vi "输入数据解析.vi"(0 "单个参数补充":dbl, 1 "从板号":dbl=1.0, 2 "主板二维码":string="BNET01", 3 "从板二维码":string="BNET01", 5 "主板引用":refnum<vi>, 7 "从板引用":refnum<vi>, 9 "主板选项":string="三级故障阀值", 11 "枚举":enum16{"主板", "从板"}(ring), 12 "快换":bool caption="快换写入") -> (4 "输出数组":dbl[][](array[numeric]), 6 "数组长度":dbl[](array[numeric]), 8 "循环次数":i32, 10 "命令":u32, 14 "名称":string[](array[string]), 15 "命令序号":u32[](array[numeric]))   [LabVIEW 2013] (continued)
                n3199 = Build Array(w8273, w8271) -> (w8272:dbl[])
              }
              frame 11 {
                # "单组温度不均衡"
                n3200 = disable-structure shown="启用" {
                  disable-tunnel: [w8288 255 ("高字节1")] -> w8284
                  disable-tunnel: w8282 -> [w8286 _]
                  frame Disabled {
                    n3201 = Unbundle By Name(w8286) -> ("单组温度不均衡"=w8285:dbl)
                    n3202 = call "输入分辨率计算-EV05.vi"("1字节?"=TRUE, "数值"=w8285, "偏移量"=0.0, "分辨率"=1.0) -> ("高字节1"=w8288:dbl)  [unwired: 1 in, 6 out]
                  }
                  frame Enabled {
                  }
                }
                n3203 = Build Array(w8284) -> (w8283:i32[])
              }
              frame 12 {
                n3204 = Unbundle By Name(w8296) -> ("SOC过高"=w8295:dbl)
                n3205 = call "输入分辨率计算-EV05.vi"("1字节?"=FALSE, "数值"=w8295, "偏移量"=0.0, "分辨率"=0.1) -> ("低字节"=w8297:dbl, "高字节1"=w8298:dbl)  [unwired: 1 in, 5 out]
                n3206 = call "二进制解析-8.6.vi"("索引"=4, "数值"=w8298) -> ("低位子数组"=w8301:i32[])  [unwired: 3 out]
                n3207 = call "二进制解析-8.6.vi"("索引"=4, "数值"=w8297) -> ("低位子数组"=w8293:i32[], "高位子数组"=w8300:i32[])  [unwired: 2 out]
                n3208 = Insert Into Array(array=w8301, new element=w8300) -> (w8299:i32[])  [unwired: 1 in]
                n3209 = call "数值二进制转十进制-8.6.vi"("子数组"=w8299) -> ("十进制数值"=w8294:i32)  [unwired: 4 out]
                n3210 = disable-structure shown="启用" {
                  disable-tunnel: w8294 -> [w8309 _]
                  disable-tunnel: [w8309 255 ("高字节1")] -> w8292
                  disable-tunnel: [w8308 i32[] [] ("低位子数组 28")] -> _
                  disable-tunnel: w8293 -> [w8308 _]
                  frame Disabled {
                  }
                  frame Enabled {
                  }
                }
                n3211 = Build Array(w8292, w8292) -> (w8305:i32[])
              }
              frame 13 {
                # "SOC过低"
                n3212 = Unbundle By Name(w8317) -> ("SOC过低"=w8316:dbl)
                n3213 = call "输入分辨率计算-EV05.vi"("1字节?"=FALSE, "数值"=w8316, "偏移量"=0.0, "分辨率"=0.1) -> ("低字节"=w8314:dbl, "高字节1"=w8315:dbl)  [unwired: 1 in, 5 out]
                n3214 = call "二进制解析-8.6.vi"("索引"=4, "数值"=w8315) -> ("低位子数组"=w8313:i32[])  [unwired: 3 out]
                n3215 = disable-structure shown="启用" {
                  disable-tunnel: w8314 -> [w8324 _]
                  disable-tunnel: [w8324 255 ("高字节1")] -> w8312
                  disable-tunnel: w8313 -> [w8323 _]
                  disable-tunnel: [w8323 i32[] [] ("低位子数组")] -> _
                  frame Disabled {
                    (unwired) i32[] [] ("低位子数组 4")
                  }
                  frame Enabled {
                  }
                }
                n3216 = Build Array(w8312, w8312) -> (w8320:i32[])
              }
              frame 14 {
                # "内阻过大"
                n3217 = disable-structure shown="启用" {
                  disable-tunnel: w8329 -> [w8334 _]
                  disable-tunnel: [w8330 255 ("高字节1")] -> w8327
                  frame Disabled {
                    n3218 = Unbundle By Name(w8334) -> ("内阻过大"=w8333:dbl)
                    n3219 = call "输入分辨率计算-EV05.vi"("1字节?"=TRUE, "数值"=w8333, "分辨率"=0.1) -> ("高字节1"=w8330:dbl)  [unwired: 2 in, 6 out]
                  }
                  frame Enabled {
                  }
                }
                n3220 = Build Array(w8327) -> (w8328:i32[])
              }
              frame 15 {
                # "极柱温度过高"
                n3221 = disable-structure shown="启用" {
                  disable-tunnel: w8338 -> [w8344 _]
                  disable-tunnel: [w8340 255 ("高字节1")] -> w8336
                  frame Disabled {
                    n3222 = Unbundle By Name(w8344) -> ("极柱温度过高"=w8343:dbl)
                    n3223 = call "输入分辨率计算-EV05.vi"("1字节?"=TRUE, "数值"=w8343, "偏移量"=-40.0, "分辨率"=1.0) -> ("高字节1"=w8340:dbl)  [unwired: 1 in, 6 out]
                  }
                  frame Enabled {
                  }
                }
                n3224 = Build Array(w8336) -> (w8337:i32[])
              }
              frame 16 {
                # "SOH过低"
                n3225 = disable-structure shown="启用" {
                  disable-tunnel: [w8361 w8369] -> w8348
                  disable-tunnel: w8347 -> [w8358 _]
                  disable-tunnel: [w8350 w8369] -> w8346
                  frame Disabled {
                    n3226 = Unbundle By Name(w8358) -> ("SOH过低"=w8357:dbl)
                    n3227 = call "输入分辨率计算-EV05.vi"("1字节?"=FALSE, "数值"=w8357, "偏移量"=0.0, "分辨率"=0.1) -> ("低字节"=w8359:dbl, "高字节1"=w8360:dbl)  [unwired: 1 in, 5 out]
                    n3228 = call "二进制解析-8.6.vi"("索引"=4, "数值"=w8360) -> ("低位子数组"=w8363:i32[])  [unwired: 3 out]
                    n3229 = call "二进制解析-8.6.vi"("索引"=4, "数值"=w8359) -> ("低位子数组"=w8352:i32[], "高位子数组"=w8362:i32[])  [unwired: 2 out]
                    n3230 = call "二进制解析-8.6.vi"("索引"=4, "数值"=0) -> ("低位子数组"=w8353:i32[])  [unwired: 3 out]
                    n3231 = Insert Into Array(array=w8363, new element=w8362) -> (w8356:i32[])  [unwired: 1 in]
                    n3232 = Insert Into Array(array=w8352, new element=w8353) -> (w8351:i32[])  [unwired: 1 in]
                    n3233 = call "数值二进制转十进制-8.6.vi"("子数组"=w8356) -> ("十进制数值"=w8361:i32)  [unwired: 4 out]
                    n3234 = call "数值二进制转十进制-8.6.vi"("子数组"=w8351) -> ("十进制数值"=w8350:i32)  [unwired: 4 out]
                  }
                  frame Enabled {
                    w8369 = 255 ("高字节1")
                  }
                }
                n3235 = Build Array(w8348, w8346) -> (w8349:i32[])
              }
            }
            n3236 = Insert Into Array(array=w8154, new element=w8155) -> (w8153:dbl[])  [unwired: 1 in]
          }
          n3237 = Build Array(w8150) -> (w8149:dbl[][])
          n3238 = Build Array("二级故障阀值") -> (w8140:string[])
        }
        frame "放电电流过高(3)" {
          n3239 = Unbundle By Name(w8375) -> ("一级故障 3"=w8376:refnum<vi>)
          n3240 = property class="Clust (严格)"(reference=w8376) -> ("Value"=w8374:T4)  [unwired: 1 in, 2 out]
          n3241 = for {
            N: 17 -> [_]
            tunnel: w8374 -> [w8386]
            shift-right: [w8383] -> w8380
            shift-left: dbl[] [] -> [w8384]
            i -> [w8387]
            n3242 = case shown="14" w8387 {
              tunnel: w8386 -> [w8388 w8399 w8410 w8420 w8430 w8440 w8452 w8464 w8476 w8488 w8500 w8512 w8526 w8547 w8559 w8568 w8577]
              tunnel: [w8389 w8400 w8411 w8421 w8431 w8442 w8454 w8466 w8478 w8490 w8502 w8513 w8535 w8550 w8558 w8567 w8579] -> w8385
              frame 0, Default {
                # "总电压过高"
                n3243 = disable-structure shown="启用" {
                  disable-tunnel: [w8395 w8398] -> w8391
                  disable-tunnel: [w8394 w8398] -> w8390
                  disable-tunnel: w8388 -> [w8393 _]
                  frame Disabled {
                    n3244 = Unbundle By Name(w8393) -> ("总电压过高"=w8392:dbl)
                    n3245 = call "输入分辨率计算-EV05.vi"("1字节?"=FALSE, "数值"=w8392, "分辨率"=0.1) -> ("低字节"=w8395:dbl, "高字节1"=w8394:dbl)  [unwired: 2 in, 5 out]
                  }
                  frame Enabled {
                    w8398 = 255 ("高字节1")
                  }
                }
                n3246 = Build Array(w8390, w8391) -> (w8389:i32[])
              }
              frame 1 {
                # "总电压过低"
                n3247 = disable-structure shown="启用" {
                  disable-tunnel: [w8406 w8409] -> w8402
                  disable-tunnel: [w8405 w8409] -> w8401
                  disable-tunnel: w8399 -> [w8404 _]
                  frame Disabled {
                    n3248 = Unbundle By Name(w8404) -> ("总电压过低"=w8403:dbl)
                    n3249 = call "输入分辨率计算-EV05.vi"("1字节?"=FALSE, "数值"=w8403, "分辨率"=0.1) -> ("低字节"=w8406:dbl, "高字节1"=w8405:dbl)  [unwired: 2 in, 5 out]
                  }
                  frame Enabled {
                    w8409 = 255 ("高字节1")
                  }
                }
                n3250 = Build Array(w8401, w8402) -> (w8400:i32[])
              }
              frame 2 {
                # "温度过高"
                n3251 = disable-structure shown="启用" {
                  disable-tunnel: [w8416 255 ("高字节1")] -> w8412
                  disable-tunnel: w8410 -> [w8414 _]
                  frame Disabled {
                    n3252 = Unbundle By Name(w8414) -> ("温度过高"=w8413:dbl)
                    n3253 = call "输入分辨率计算-EV05.vi"("1字节?"=TRUE, "数值"=w8413, "偏移量"=-40.0, "分辨率"=1.0) -> ("高字节1"=w8416:dbl)  [unwired: 1 in, 6 out]
                  }
                  frame Enabled {
                  }
                }
                n3254 = Build Array(w8412) -> (w8411:i32[])
              }
              frame 3 {
                # "温度过低"
                n3255 = disable-structure shown="启用" {
                  disable-tunnel: [w8426 255 ("高字节1")] -> w8422
                  disable-tunnel: w8420 -> [w8424 _]
                  frame Disabled {
                    n3256 = Unbundle By Name(w8424) -> ("温度过低"=w8423:dbl)
                    n3257 = call "输入分辨率计算-EV05.vi"("1字节?"=TRUE, "数值"=w8423, "偏移量"=-40.0, "分辨率"=1.0) -> ("高字节1"=w8426:dbl)  [unwired: 1 in, 6 out]
                  }
                  frame Enabled {
                  }
                }
                n3258 = Build Array(w8422) -> (w8421:i32[])
              }
              frame 4 {
                # "整组温度不均衡"
                n3259 = disable-structure shown="启用" {
                  disable-tunnel: [w8436 255 ("高字节1")] -> w8432
                  disable-tunnel: w8430 -> [w8434 _]
                  frame Disabled {
                    n3260 = Unbundle By Name(w8434) -> ("整组温度不均衡"=w8433:dbl)
                    n3261 = call "输入分辨率计算-EV05.vi"("1字节?"=TRUE, "数值"=w8433, "偏移量"=0.0, "分辨率"=1.0) -> ("高字节1"=w8436:dbl)  [unwired: 1 in, 6 out]
                  }
                  frame Enabled {
                  }
                }
                n3262 = Build Array(w8432) -> (w8431:i32[])
              }
              frame 5 {
                # "单组电压不均衡"
                n3263 = disable-structure shown="启用" {
                  disable-tunnel: [w8448 w8451] -> w8443
                  disable-tunnel: [w8446 w8451] -> w8441
                  disable-tunnel: w8440 -> [w8445 _]
                  frame Disabled {
                    n3264 = Unbundle By Name(w8445) -> ("单组电压不均衡"=w8444:dbl)
                    n3265 = call "输入分辨率计算-EV05.vi"("1字节?"=FALSE, "数值"=w8444, "偏移量"=0.0, "分辨率"=0.001) -> ("低字节"=w8446:dbl, "高字节1"=w8448:dbl)  [unwired: 1 in, 5 out]
                  }
                  frame Enabled {
                    w8451 = 255 ("高字节1")
                  }
                }
                n3266 = Build Array(w8443, w8441) -> (w8442:i32[])
              }
              frame 6 {
                # "整组电压不均衡"
                n3267 = disable-structure shown="启用" {
                  disable-tunnel: [w8460 w8463] -> w8455
                  disable-tunnel: [w8458 w8463] -> w8453
                  disable-tunnel: w8452 -> [w8457 _]
                  frame Disabled {
                    n3268 = Unbundle By Name(w8457) -> ("整组电压不均衡"=w8456:dbl)
                    n3269 = call "输入分辨率计算-EV05.vi"("1字节?"=FALSE, "数值"=w8456, "偏移量"=0.0, "分辨率"=0.001) -> ("低字节"=w8458:dbl, "高字节1"=w8460:dbl)  [unwired: 1 in, 5 out]
                  }
                  frame Enabled {
                    w8463 = 255 ("高字节1")
                  }
                }
                n3270 = Build Array(w8455, w8453) -> (w8454:i32[])
              }
              frame 7 {
                # "单体电压过高"
                n3271 = disable-structure shown="启用" {
                  disable-tunnel: [w8472 w8475] -> w8467
                  disable-tunnel: [w8470 w8475] -> w8465
                  disable-tunnel: w8464 -> [w8469 _]
                  frame Disabled {
                    n3272 = Unbundle By Name(w8469) -> ("单体电压过高"=w8468:dbl)
                    n3273 = call "输入分辨率计算-EV05.vi"("1字节?"=FALSE, "数值"=w8468, "偏移量"=0.0, "分辨率"=0.001) -> ("低字节"=w8470:dbl, "高字节1"=w8472:dbl)  [unwired: 1 in, 5 out]
                  }
                  frame Enabled {
                    w8475 = 255 ("高字节1")
                  }
                }
                n3274 = Build Array(w8467, w8465) -> (w8466:i32[])
              }
              frame 8 {
                # "单体电压过低"
                n3275 = disable-structure shown="启用" {
                  disable-tunnel: [w8484 w8487] -> w8479
                  disable-tunnel: [w8482 w8487] -> w8477
                  disable-tunnel: w8476 -> [w8481 _]
                  frame Disabled {
                    n3276 = Unbundle By Name(w8481) -> ("单体电压过低"=w8480:dbl)
                    n3277 = call "输入分辨率计算-EV05.vi"("1字节?"=FALSE, "数值"=w8480, "偏移量"=0.0, "分辨率"=0.001) -> ("低字节"=w8482:dbl, "高字节1"=w8484:dbl)  [unwired: 1 in, 5 out]
                  }
                  frame Enabled {
                    w8487 = 255 ("高字节1")
                  }
                }
                n3278 = Build Array(w8479, w8477) -> (w8478:i32[])
              }
              frame 9 {
                # "充电电流过高"
                n3279 = disable-structure shown="启用" {
                  disable-tunnel: [w8496 w8499] -> w8491
                  disable-tunnel: [w8494 w8499] -> w8489
                  disable-tunnel: w8488 -> [w8493 _]
                  frame Disabled {
                    n3280 = Unbundle By Name(w8493) -> ("充电电流过高"=w8492:dbl)
                    n3281 = call "输入分辨率计算-EV05.vi"("1字节?"=FALSE, "数值"=w8492, "偏移量"=-3000.0, "分辨率"=0.1) -> ("低字节"=w8494:dbl, "高字节1"=w8496:dbl)  [unwired: 1 in, 5 out]
                  }
                  frame Enabled {
                    w8499 = 255 ("高字节1")
                  }
                }
                n3282 = Build Array(w8491, w8489) -> (w8490:i32[])
              }
              frame 10 {
                # "放电电流过高"
                n3283 = disable-structure shown="启用" {
                  disable-tunnel: [w8508 w8511] -> w8503
                  disable-tunnel: [w8506 w8511] -> w8501
                  disable-tunnel: w8500 -> [w8505 _]
                  frame Enabled {
                    n3284 = Unbundle By Name(w8505) -> ("放电电流过高"=w8504:dbl)
                    n3285 = call "输入分辨率计算-EV05.vi"("1字节?"=FALSE, "数值"=w8504, "偏移量"=0.0, "分辨率"=0.1) -> ("低字节"=w8506:dbl, "高字节1"=w8508:dbl)  [unwired: 1 in, 5 out]
                  }
                  frame Disabled {
                    w8511 = 255 ("高字节1")
                  }
                }
                n3286 = Build Array(w8503, w8501) -> (w8502:dbl[])
              }
              frame 11 {
                # "单组温度不均衡"
                n3287 = disable-structure shown="启用" {
                  disable-tunnel: [w8518 255 ("高字节1")] -> w8514
                  disable-tunnel: w8512 -> [w8516 _]
                  frame Disabled {
                    n3288 = Unbundle By Name(w8516) -> ("单组温度不均衡"=w8515:dbl)
                    n3289 = call "输入分辨率计算-EV05.vi"("1字节?"=TRUE, "数值"=w8515, "偏移量"=0.0, "分辨率"=1.0) -> ("高字节1"=w8518:dbl)  [unwired: 1 in, 6 out]
                  }
                  frame Enabled {
                  }
                }
                n3290 = Build Array(w8514) -> (w8513:i32[])
              }
              frame 12 {
                # "SOC过高"
                n3291 = Unbundle By Name(w8526) -> ("SOC过高"=w8525:dbl)
                n3292 = call "输入分辨率计算-EV05.vi"("1字节?"=FALSE, "数值"=w8525, "偏移量"=0.0, "分辨率"=0.1) -> ("低字节"=w8527:dbl, "高字节1"=w8528:dbl)  [unwired: 1 in, 5 out]
                n3293 = call "二进制解析-8.6.vi"("索引"=4, "数值"=w8528) -> ("低位子数组"=w8531:i32[])  [unwired: 3 out]
                n3294 = call "二进制解析-8.6.vi"("索引"=4, "数值"=w8527) -> ("低位子数组"=w8523:i32[], "高位子数组"=w8530:i32[])  [unwired: 2 out]
                n3295 = Insert Into Array(array=w8531, new element=w8530) -> (w8529:i32[])  [unwired: 1 in]
                n3296 = call "数值二进制转十进制-8.6.vi"("子数组"=w8529) -> ("十进制数值"=w8524:i32)  [unwired: 4 out]
                n3297 = disable-structure shown="启用" {
                  disable-tunnel: w8524 -> [w8539 _]
                  disable-tunnel: [w8539 255 ("高字节1")] -> w8522
                  disable-tunnel: [w8538 i32[] [] ("低位子数组 28")] -> _
                  disable-tunnel: w8523 -> [w8538 _]
                  frame Disabled {
                  }
                  frame Enabled {
                  }
                }
                n3298 = Build Array(w8522, w8522) -> (w8535:i32[])
              }
              frame 13 {
                # "SOC过低"
                n3299 = Unbundle By Name(w8547) -> ("SOC过低"=w8546:dbl)
                n3300 = call "输入分辨率计算-EV05.vi"("1字节?"=FALSE, "数值"=w8546, "偏移量"=0.0, "分辨率"=0.1) -> ("低字节"=w8544:dbl, "高字节1"=w8545:dbl)  [unwired: 1 in, 5 out]
                n3301 = call "二进制解析-8.6.vi"("索引"=4, "数值"=w8545) -> ("低位子数组"=w8543:i32[])  [unwired: 3 out]
                n3302 = disable-structure shown="启用" {
                  disable-tunnel: w8544 -> [w8554 _]
                  disable-tunnel: [w8554 255 ("高字节1")] -> w8542
                  disable-tunnel: w8543 -> [w8553 _]
                  disable-tunnel: [w8553 i32[] [] ("低位子数组")] -> _
                  frame Disabled {
                    (unwired) i32[] [] ("低位子数组 4")
                  }
                  frame Enabled {
                  }
                }
                n3303 = Build Array(w8542, w8542) -> (w8550:i32[])
              }
              frame 14 {
                # "内阻过大"
                n3304 = disable-structure shown="启用" {
                  disable-tunnel: w8559 -> [w8564 _]
                  disable-tunnel: [w8560 255 ("高字节1")] -> w8557
                  frame Disabled {
                    n3305 = Unbundle By Name(w8564) -> ("内阻过大"=w8563:dbl)
                    n3306 = call "输入分辨率计算-EV05.vi"("1字节?"=TRUE, "数值"=w8563, "分辨率"=0.1) -> ("高字节1"=w8560:dbl)  [unwired: 2 in, 6 out]
                  }
                  frame Enabled {
                  }
                }
                n3307 = Build Array(w8557) -> (w8558:i32[])
              }
              frame 15 {
                # "极柱温度过高"
                n3308 = disable-structure shown="启用" {
                  disable-tunnel: w8568 -> [w8574 _]
                  disable-tunnel: [w8570 255 ("高字节1")] -> w8566
                  frame Disabled {
                    n3309 = Unbundle By Name(w8574) -> ("极柱温度过高"=w8573:dbl)
                    n3310 = call "输入分辨率计算-EV05.vi"("1字节?"=TRUE, "数值"=w8573, "偏移量"=-40.0, "分辨率"=1.0) -> ("高字节1"=w8570:dbl)  [unwired: 1 in, 6 out]
                  }
                  frame Enabled {
                  }
                }
                n3311 = Build Array(w8566) -> (w8567:i32[])
              }
              frame 16 {
                # "SOH过低"
                n3312 = disable-structure shown="启用" {
                  disable-tunnel: [w8591 w8599] -> w8578
                  disable-tunnel: w8577 -> [w8588 _]
                  disable-tunnel: [w8580 w8599] -> w8576
                  frame Disabled {
                    n3313 = Unbundle By Name(w8588) -> ("SOH过低"=w8587:dbl)
                    n3314 = call "输入分辨率计算-EV05.vi"("1字节?"=FALSE, "数值"=w8587, "偏移量"=0.0, "分辨率"=0.1) -> ("低字节"=w8589:dbl, "高字节1"=w8590:dbl)  [unwired: 1 in, 5 out]
                    n3315 = call "二进制解析-8.6.vi"("索引"=4, "数值"=w8590) -> ("低位子数组"=w8593:i32[])  [unwired: 3 out]
                    n3316 = call "二进制解析-8.6.vi"("索引"=4, "数值"=w8589) -> ("低位子数组"=w8582:i32[], "高位子数组"=w8592:i32[])  [unwired: 2 out]
                    n3317 = call "二进制解析-8.6.vi"("索引"=4, "数值"=0) -> ("低位子数组"=w8583:i32[])  [unwired: 3 out]
                    n3318 = Insert Into Array(array=w8593, new element=w8592) -> (w8586:i32[])  [unwired: 1 in]
                    n3319 = Insert Into Array(array=w8582, new element=w8583) -> (w8581:i32[])  [unwired: 1 in]
                    n3320 = call "数值二进制转十进制-8.6.vi"("子数组"=w8586) -> ("十进制数值"=w8591:i32)  [unwired: 4 out]
                    n3321 = call "数值二进制转十进制-8.6.vi"("子数组"=w8581) -> ("十进制数值"=w8580:i32)  [unwired: 4 out]
                  }
                  frame Enabled {
                    w8599 = 255 ("高字节1")
                  }
                }
                n3322 = Build Array(w8578, w8576) -> (w8579:i32[])
              }
            }
            n3323 = Insert Into Array(array=w8384, new element=w8385) -> (w8383:dbl[])  [unwired: 1 in]
          }
          n3324 = Build Array(w8380) -> (w8379:dbl[][])
          n3325 = Build Array("三级故障阀值") -> (w8370:string[])
        }
        frame "单组温度不均衡" {
          n3326 = Unbundle By Name(w8605) -> ("一级故障"=w8606:refnum<vi>)
          n3327 = property class="Clust (严格)"(reference=w8606) -> ("Value"=w8604:T4)  [unwired: 1 in, 2 out]
          n3328 = for {
            N: 17 -> [_]
            tunnel: w8604 -> [w8616]
            shift-right: [w8613] -> w8610
            shift-left: dbl[] [] -> [w8614]
            i -> [w8617]
            n3329 = case shown="11" w8617 {
              tunnel: w8616 -> [w8618 w8629 w8640 w8650 w8660 w8670 w8682 w8694 w8706 w8718 w8730 w8742 w8755 w8776 w8788 w8797 w8806]
              tunnel: [w8619 w8630 w8641 w8651 w8661 w8672 w8684 w8696 w8708 w8720 w8732 w8743 w8764 w8779 w8787 w8796 w8808] -> w8615
              frame 0, Default {
                # "总电压过高"
                n3330 = disable-structure shown="启用" {
                  disable-tunnel: [w8625 w8628] -> w8621
                  disable-tunnel: [w8624 w8628] -> w8620
                  disable-tunnel: w8618 -> [w8623 _]
                  frame Disabled {
                    n3331 = Unbundle By Name(w8623) -> ("总电压过高"=w8622:dbl)
                    n3332 = call "输入分辨率计算-EV05.vi"("1字节?"=FALSE, "数值"=w8622, "分辨率"=0.1) -> ("低字节"=w8625:dbl, "高字节1"=w8624:dbl)  [unwired: 2 in, 5 out]
                  }
                  frame Enabled {
                    w8628 = 255 ("高字节1")
                  }
                }
                n3333 = Build Array(w8620, w8621) -> (w8619:i32[])
              }
              frame 1 {
                # "总电压过低"
                n3334 = disable-structure shown="启用" {
                  disable-tunnel: [w8636 w8639] -> w8632
                  disable-tunnel: [w8635 w8639] -> w8631
                  disable-tunnel: w8629 -> [w8634 _]
                  frame Disabled {
                    n3335 = Unbundle By Name(w8634) -> ("总电压过低"=w8633:dbl)
                    n3336 = call "输入分辨率计算-EV05.vi"("1字节?"=FALSE, "数值"=w8633, "分辨率"=0.1) -> ("低字节"=w8636:dbl, "高字节1"=w8635:dbl)  [unwired: 2 in, 5 out]
                  }
                  frame Enabled {
                    w8639 = 255 ("高字节1")
                  }
                }
                n3337 = Build Array(w8631, w8632) -> (w8630:i32[])
              }
              frame 2 {
                # "温度过高"
                n3338 = disable-structure shown="启用" {
                  disable-tunnel: [w8646 255 ("高字节1")] -> w8642
                  disable-tunnel: w8640 -> [w8644 _]
                  frame Disabled {
                    n3339 = Unbundle By Name(w8644) -> ("温度过高"=w8643:dbl)
                    n3340 = call "输入分辨率计算-EV05.vi"("1字节?"=TRUE, "数值"=w8643, "偏移量"=-40.0, "分辨率"=1.0) -> ("高字节1"=w8646:dbl)  [unwired: 1 in, 6 out]
                  }
                  frame Enabled {
                  }
                }
                n3341 = Build Array(w8642) -> (w8641:i32[])
              }
              frame 3 {
                # "温度过低"
                n3342 = disable-structure shown="启用" {
                  disable-tunnel: [w8656 255 ("高字节1")] -> w8652
                  disable-tunnel: w8650 -> [w8654 _]
                  frame Disabled {
                    n3343 = Unbundle By Name(w8654) -> ("温度过低"=w8653:dbl)
                    n3344 = call "输入分辨率计算-EV05.vi"("1字节?"=TRUE, "数值"=w8653, "偏移量"=-40.0, "分辨率"=1.0) -> ("高字节1"=w8656:dbl)  [unwired: 1 in, 6 out]
                  }
                  frame Enabled {
                  }
                }
                n3345 = Build Array(w8652) -> (w8651:i32[])
              }
              frame 4 {
                # "整组温度不均衡"
                n3346 = disable-structure shown="启用" {
                  disable-tunnel: [w8666 255 ("高字节1")] -> w8662
                  disable-tunnel: w8660 -> [w8664 _]
                  frame Disabled {
                    n3347 = Unbundle By Name(w8664) -> ("整组温度不均衡"=w8663:dbl)
                    n3348 = call "输入分辨率计算-EV05.vi"("1字节?"=TRUE, "数值"=w8663, "偏移量"=0.0, "分辨率"=1.0) -> ("高字节1"=w8666:dbl)  [unwired: 1 in, 6 out]
                  }
                  frame Enabled {
                  }
                }
                n3349 = Build Array(w8662) -> (w8661:i32[])
              }
              frame 5 {
                # "单组电压不均衡"
                n3350 = disable-structure shown="启用" {
                  disable-tunnel: [w8678 w8681] -> w8673
                  disable-tunnel: [w8676 w8681] -> w8671
                  disable-tunnel: w8670 -> [w8675 _]
                  frame Disabled {
                    n3351 = Unbundle By Name(w8675) -> ("单组电压不均衡"=w8674:dbl)
                    n3352 = call "输入分辨率计算-EV05.vi"("1字节?"=FALSE, "数值"=w8674, "偏移量"=0.0, "分辨率"=0.001) -> ("低字节"=w8676:dbl, "高字节1"=w8678:dbl)  [unwired: 1 in, 5 out]
                  }
                  frame Enabled {
                    w8681 = 255 ("高字节1")
                  }
                }
                n3353 = Build Array(w8673, w8671) -> (w8672:i32[])
              }
              frame 6 {
                # "整组电压不均衡"
                n3354 = disable-structure shown="启用" {
                  disable-tunnel: [w8690 w8693] -> w8685
                  disable-tunnel: [w8688 w8693] -> w8683
                  disable-tunnel: w8682 -> [w8687 _]
                  frame Disabled {
                    n3355 = Unbundle By Name(w8687) -> ("整组电压不均衡"=w8686:dbl)
                    n3356 = call "输入分辨率计算-EV05.vi"("1字节?"=FALSE, "数值"=w8686, "偏移量"=0.0, "分辨率"=0.001) -> ("低字节"=w8688:dbl, "高字节1"=w8690:dbl)  [unwired: 1 in, 5 out]
                  }
                  frame Enabled {
                    w8693 = 255 ("高字节1")
                  }
                }
                n3357 = Build Array(w8685, w8683) -> (w8684:i32[])
              }
              frame 7 {
                # "单体电压过高"
                n3358 = disable-structure shown="启用" {
                  disable-tunnel: [w8702 w8705] -> w8697
                  disable-tunnel: [w8700 w8705] -> w8695
                  disable-tunnel: w8694 -> [w8699 _]
                  frame Disabled {
                    n3359 = Unbundle By Name(w8699) -> ("单体电压过高"=w8698:dbl)
                    n3360 = call "输入分辨率计算-EV05.vi"("1字节?"=FALSE, "数值"=w8698, "偏移量"=0.0, "分辨率"=0.001) -> ("低字节"=w8700:dbl, "高字节1"=w8702:dbl)  [unwired: 1 in, 5 out]
                  }
                  frame Enabled {
                    w8705 = 255 ("高字节1")
                  }
                }
                n3361 = Build Array(w8697, w8695) -> (w8696:i32[])
              }
              frame 8 {
                # "单体电压过低"
                n3362 = disable-structure shown="启用" {
                  disable-tunnel: [w8714 w8717] -> w8709
                  disable-tunnel: [w8712 w8717] -> w8707
                  disable-tunnel: w8706 -> [w8711 _]
                  frame Disabled {
                    n3363 = Unbundle By Name(w8711) -> ("单体电压过低"=w8710:dbl)
                    n3364 = call "输入分辨率计算-EV05.vi"("1字节?"=FALSE, "数值"=w8710, "偏移量"=0.0, "分辨率"=0.001) -> ("低字节"=w8712:dbl, "高字节1"=w8714:dbl)  [unwired: 1 in, 5 out]
                  }
                  frame Enabled {
                    w8717 = 255 ("高字节1")
                  }
                }
                n3365 = Build Array(w8709, w8707) -> (w8708:i32[])
              }
              frame 9 {
                # "充电电流过高"
                n3366 = disable-structure shown="启用" {
                  disable-tunnel: [w8726 w8729] -> w8721
                  disable-tunnel: [w8724 w8729] -> w8719
                  disable-tunnel: w8718 -> [w8723 _]
                  frame Disabled {
                    n3367 = Unbundle By Name(w8723) -> ("充电电流过高"=w8722:dbl)
                    n3368 = call "输入分辨率计算-EV05.vi"("1字节?"=FALSE, "数值"=w8722, "偏移量"=-3000.0, "分辨率"=0.1) -> ("低字节"=w8724:dbl, "高字节1"=w8726:dbl)  [unwired: 1 in, 5 out]
                  }
                  frame Enabled {
                    w8729 = 255 ("高字节1")
                  }
                }
                n3369 = Build Array(w8721, w8719) -> (w8720:i32[])
              }
              frame 10 {
                # "放电电流过高"
                n3370 = disable-structure shown="启用" {
                  disable-tunnel: [w8738 w8741] -> w8733
                  disable-tunnel: [w8736 w8741] -> w8731
                  disable-tunnel: w8730 -> [w8735 _]
                  frame Disabled {
                    n3371 = Unbundle By Name(w8735) -> ("放电电流过高"=w8734:dbl)
                    n3372 = call "输入分辨率计算-EV05.vi"("1字节?"=FALSE, "数值"=w8734, "偏移量"=-3000.0, "分辨率"=0.1) -> ("低字节"=w8736:dbl, "高字节1"=w8738:dbl)  [unwired: 1 in, 5 out]
                  }
                  frame Enabled {
                    w8741 = 255 ("高字节1")
                  }
                }
                n3373 = Build Array(w8733, w8731) -> (w8732:i32[])
              }
              frame 11 {
                # "单组温度不均衡"
                n3374 = disable-structure shown="启用" {
                  disable-tunnel: [w8747 255 ("高字节1")] -> w8744
                  disable-tunnel: w8742 -> [w8746 _]
                  frame Enabled {
                    n3375 = Unbundle By Name(w8746) -> ("单组温度不均衡"=w8745:dbl)
                    n3376 = call "输入分辨率计算-EV05.vi"("1字节?"=TRUE, "数值"=w8745, "分辨率"=1.0) -> ("高字节1"=w8747:dbl)  [unwired: 2 in, 6 out]
                  }
                  frame Disabled {
                  }
                }
                n3377 = Build Array(w8744) -> (w8743:dbl[])
              }
              frame 12 {
                # "SOC过高"
                n3378 = Unbundle By Name(w8755) -> ("SOC过高"=w8754:dbl)
                n3379 = call "输入分辨率计算-EV05.vi"("1字节?"=FALSE, "数值"=w8754, "偏移量"=0.0, "分辨率"=0.1) -> ("低字节"=w8756:dbl, "高字节1"=w8757:dbl)  [unwired: 1 in, 5 out]
                n3380 = call "二进制解析-8.6.vi"("索引"=4, "数值"=w8757) -> ("低位子数组"=w8760:i32[])  [unwired: 3 out]
                n3381 = call "二进制解析-8.6.vi"("索引"=4, "数值"=w8756) -> ("低位子数组"=w8752:i32[], "高位子数组"=w8759:i32[])  [unwired: 2 out]
                n3382 = Insert Into Array(array=w8760, new element=w8759) -> (w8758:i32[])  [unwired: 1 in]
                n3383 = call "数值二进制转十进制-8.6.vi"("子数组"=w8758) -> ("十进制数值"=w8753:i32)  [unwired: 4 out]
                n3384 = disable-structure shown="启用" {
                  disable-tunnel: w8753 -> [w8768 _]
                  disable-tunnel: [w8768 255 ("高字节1")] -> w8751
                  disable-tunnel: w8752 -> [w8767 _]
                  disable-tunnel: [w8767 i32[] [] ("低位子数组 29")] -> _
                  frame Disabled {
                  }
                  frame Enabled {
                  }
                }
                n3385 = Build Array(w8751, w8751) -> (w8764:i32[])
              }
              frame 13 {
                # "SOC过低"
                n3386 = Unbundle By Name(w8776) -> ("SOC过低"=w8775:dbl)
                n3387 = call "输入分辨率计算-EV05.vi"("1字节?"=FALSE, "数值"=w8775, "偏移量"=0.0, "分辨率"=0.1) -> ("低字节"=w8773:dbl, "高字节1"=w8774:dbl)  [unwired: 1 in, 5 out]
                n3388 = call "二进制解析-8.6.vi"("索引"=4, "数值"=w8774) -> ("低位子数组"=w8772:i32[])  [unwired: 3 out]
                n3389 = disable-structure shown="启用" {
                  disable-tunnel: w8773 -> [w8783 _]
                  disable-tunnel: [w8783 255 ("高字节1")] -> w8771
                  disable-tunnel: w8772 -> [w8782 _]
                  disable-tunnel: [w8782 i32[] [] ("低位子数组")] -> _
                  frame Disabled {
                    (unwired) i32[] [] ("低位子数组 4")
                  }
                  frame Enabled {
                  }
                }
                n3390 = Build Array(w8771, w8771) -> (w8779:i32[])
              }
              frame 14 {
                # "内阻过大"
                n3391 = disable-structure shown="启用" {
                  disable-tunnel: w8788 -> [w8793 _]
                  disable-tunnel: [w8789 255 ("高字节1")] -> w8786
                  frame Disabled {
                    n3392 = Unbundle By Name(w8793) -> ("内阻过大"=w8792:dbl)
                    n3393 = call "输入分辨率计算-EV05.vi"("1字节?"=TRUE, "数值"=w8792, "分辨率"=0.1) -> ("高字节1"=w8789:dbl)  [unwired: 2 in, 6 out]
                  }
                  frame Enabled {
                  }
                }
                n3394 = Build Array(w8786) -> (w8787:i32[])
              }
              frame 15 {
                # "极柱温度过高"
                n3395 = disable-structure shown="启用" {
                  disable-tunnel: w8797 -> [w8803 _]
                  disable-tunnel: [w8799 255 ("高字节1")] -> w8795
                  frame Disabled {
                    n3396 = Unbundle By Name(w8803) -> ("极柱温度过高"=w8802:dbl)
                    n3397 = call "输入分辨率计算-EV05.vi"("1字节?"=TRUE, "数值"=w8802, "偏移量"=-40.0, "分辨率"=1.0) -> ("高字节1"=w8799:dbl)  [unwired: 1 in, 6 out]
                  }
                  frame Enabled {
                  }
                }
                n3398 = Build Array(w8795) -> (w8796:i32[])
              }
              frame 16 {
                # "SOH过低"
                n3399 = disable-structure shown="启用" {
                  disable-tunnel: [w8820 w8828] -> w8807
                  disable-tunnel: w8806 -> [w8817 _]
                  disable-tunnel: [w8809 w8828] -> w8805
                  frame Disabled {
                    n3400 = Unbundle By Name(w8817) -> ("SOH过低"=w8816:dbl)
                    n3401 = call "输入分辨率计算-EV05.vi"("1字节?"=FALSE, "数值"=w8816, "偏移量"=0.0, "分辨率"=0.1) -> ("低字节"=w8818:dbl, "高字节1"=w8819:dbl)  [unwired: 1 in, 5 out]
                    n3402 = call "二进制解析-8.6.vi"("索引"=4, "数值"=w8819) -> ("低位子数组"=w8822:i32[])  [unwired: 3 out]
                    n3403 = call "二进制解析-8.6.vi"("索引"=4, "数值"=w8818) -> ("低位子数组"=w8811:i32[], "高位子数组"=w8821:i32[])  [unwired: 2 out]
                    n3404 = call "二进制解析-8.6.vi"("索引"=4, "数值"=0) -> ("低位子数组"=w8812:i32[])  [unwired: 3 out]
                    n3405 = Insert Into Array(array=w8822, new element=w8821) -> (w8815:i32[])  [unwired: 1 in]
                    n3406 = Insert Into Array(array=w8811, new element=w8812) -> (w8810:i32[])  [unwired: 1 in]
                    n3407 = call "数值二进制转十进制-8.6.vi"("子数组"=w8815) -> ("十进制数值"=w8820:i32)  [unwired: 4 out]
                    n3408 = call "数值二进制转十进制-8.6.vi"("子数组"=w8810) -> ("十进制数值"=w8809:i32)  [unwired: 4 out]
                  }
                  frame Enabled {
                    w8828 = 255 ("高字节1")
                  }
                }
                n3409 = Build Array(w8807, w8805) -> (w8808:i32[])
              }
            }
            n3410 = Insert Into Array(array=w8614, new element=w8615) -> (w8613:dbl[])  [unwired: 1 in]
          }
          n3411 = Build Array(w8610) -> (w8609:dbl[][])
          n3412 = Build Array("一级故障阀值") -> (w8600:string[])
        }
        frame "单组温度不均衡(2)" {
          n3413 = Unbundle By Name(w8834) -> ("一级故障 2"=w8835:refnum<vi>)
          n3414 = property class="Clust (严格)"(reference=w8835) -> ("Value"=w8833:T4)  [unwired: 1 in, 2 out]
          n3415 = for {
            N: 17 -> [_]
            tunnel: w8833 -> [w8845]
            shift-right: [w8842] -> w8839
            shift-left: dbl[] [] -> [w8843]
            i -> [w8846]
            n3416 = case shown="11" w8846 {
              tunnel: w8845 -> [w8847 w8858 w8869 w8879 w8889 w8899 w8911 w8923 w8935 w8947 w8959 w8971 w8984 w9005 w9017 w9026 w9035]
              tunnel: [w8848 w8859 w8870 w8880 w8890 w8901 w8913 w8925 w8937 w8949 w8961 w8972 w8993 w9008 w9016 w9025 w9037] -> w8844
              frame 0, Default {
                # "总电压过高"
                n3417 = disable-structure shown="启用" {
                  disable-tunnel: [w8854 w8857] -> w8850
                  disable-tunnel: [w8853 w8857] -> w8849
                  disable-tunnel: w8847 -> [w8852 _]
                  frame Disabled {
                    n3418 = Unbundle By Name(w8852) -> ("总电压过高"=w8851:dbl)
                    n3419 = call "输入分辨率计算-EV05.vi"("1字节?"=FALSE, "数值"=w8851, "分辨率"=0.1) -> ("低字节"=w8854:dbl, "高字节1"=w8853:dbl)  [unwired: 2 in, 5 out]
                  }
                  frame Enabled {
                    w8857 = 255 ("高字节1")
                  }
                }
                n3420 = Build Array(w8849, w8850) -> (w8848:i32[])
              }
              frame 1 {
                # "总电压过低"
                n3421 = disable-structure shown="启用" {
                  disable-tunnel: [w8865 w8868] -> w8861
                  disable-tunnel: [w8864 w8868] -> w8860
                  disable-tunnel: w8858 -> [w8863 _]
                  frame Disabled {
                    n3422 = Unbundle By Name(w8863) -> ("总电压过低"=w8862:dbl)
                    n3423 = call "输入分辨率计算-EV05.vi"("1字节?"=FALSE, "数值"=w8862, "分辨率"=0.1) -> ("低字节"=w8865:dbl, "高字节1"=w8864:dbl)  [unwired: 2 in, 5 out]
                  }
                  frame Enabled {
                    w8868 = 255 ("高字节1")
                  }
                }
                n3424 = Build Array(w8860, w8861) -> (w8859:i32[])
              }
              frame 2 {
                # "温度过高"
                n3425 = disable-structure shown="启用" {
                  disable-tunnel: [w8875 255 ("高字节1")] -> w8871
                  disable-tunnel: w8869 -> [w8873 _]
                  frame Disabled {
                    n3426 = Unbundle By Name(w8873) -> ("温度过高"=w8872:dbl)
                    n3427 = call "输入分辨率计算-EV05.vi"("1字节?"=TRUE, "数值"=w8872, "偏移量"=-40.0, "分辨率"=1.0) -> ("高字节1"=w8875:dbl)  [unwired: 1 in, 6 out]
                  }
                  frame Enabled {
                  }
                }
                n3428 = Build Array(w8871) -> (w8870:i32[])
              }
              frame 3 {
                # "温度过低"
                n3429 = disable-structure shown="启用" {
                  disable-tunnel: [w8885 255 ("高字节1")] -> w8881
                  disable-tunnel: w8879 -> [w8883 _]
                  frame Disabled {
                    n3430 = Unbundle By Name(w8883) -> ("温度过低"=w8882:dbl)
                    n3431 = call "输入分辨率计算-EV05.vi"("1字节?"=TRUE, "数值"=w8882, "偏移量"=-40.0, "分辨率"=1.0) -> ("高字节1"=w8885:dbl)  [unwired: 1 in, 6 out]
                  }
                  frame Enabled {
                  }
                }
                n3432 = Build Array(w8881) -> (w8880:i32[])
              }
              frame 4 {
                # "整组温度不均衡"
                n3433 = disable-structure shown="启用" {
                  disable-tunnel: [w8895 255 ("高字节1")] -> w8891
                  disable-tunnel: w8889 -> [w8893 _]
                  frame Disabled {
                    n3434 = Unbundle By Name(w8893) -> ("整组温度不均衡"=w8892:dbl)
                    n3435 = call "输入分辨率计算-EV05.vi"("1字节?"=TRUE, "数值"=w8892, "偏移量"=0.0, "分辨率"=1.0) -> ("高字节1"=w8895:dbl)  [unwired: 1 in, 6 out]
                  }
                  frame Enabled {
                  }
                }
                n3436 = Build Array(w8891) -> (w8890:i32[])
              }
              frame 5 {
                # "单组电压不均衡"
                n3437 = disable-structure shown="启用" {
                  disable-tunnel: [w8907 w8910] -> w8902
                  disable-tunnel: [w8905 w8910] -> w8900
                  disable-tunnel: w8899 -> [w8904 _]
                  frame Disabled {
                    n3438 = Unbundle By Name(w8904) -> ("单组电压不均衡"=w8903:dbl)
                    n3439 = call "输入分辨率计算-EV05.vi"("1字节?"=FALSE, "数值"=w8903, "偏移量"=0.0, "分辨率"=0.001) -> ("低字节"=w8905:dbl, "高字节1"=w8907:dbl)  [unwired: 1 in, 5 out]
                  }
                  frame Enabled {
                    w8910 = 255 ("高字节1")
                  }
                }
                n3440 = Build Array(w8902, w8900) -> (w8901:i32[])
              }
              frame 6 {
                # "整组电压不均衡"
                n3441 = disable-structure shown="启用" {
                  disable-tunnel: [w8919 w8922] -> w8914
                  disable-tunnel: [w8917 w8922] -> w8912
                  disable-tunnel: w8911 -> [w8916 _]
                  frame Disabled {
                    n3442 = Unbundle By Name(w8916) -> ("整组电压不均衡"=w8915:dbl)
                    n3443 = call "输入分辨率计算-EV05.vi"("1字节?"=FALSE, "数值"=w8915, "偏移量"=0.0, "分辨率"=0.001) -> ("低字节"=w8917:dbl, "高字节1"=w8919:dbl)  [unwired: 1 in, 5 out]
                  }
                  frame Enabled {
                    w8922 = 255 ("高字节1")
                  }
                }
                n3444 = Build Array(w8914, w8912) -> (w8913:i32[])
              }
              frame 7 {
                # "单体电压过高"
                n3445 = disable-structure shown="启用" {
                  disable-tunnel: [w8931 w8934] -> w8926
                  disable-tunnel: [w8929 w8934] -> w8924
                  disable-tunnel: w8923 -> [w8928 _]
                  frame Disabled {
                    n3446 = Unbundle By Name(w8928) -> ("单体电压过高"=w8927:dbl)
                    n3447 = call "输入分辨率计算-EV05.vi"("1字节?"=FALSE, "数值"=w8927, "偏移量"=0.0, "分辨率"=0.001) -> ("低字节"=w8929:dbl, "高字节1"=w8931:dbl)  [unwired: 1 in, 5 out]
                  }
                  frame Enabled {
                    w8934 = 255 ("高字节1")
                  }
                }
                n3448 = Build Array(w8926, w8924) -> (w8925:i32[])
              }
              frame 8 {
                # "单体电压过低"
                n3449 = disable-structure shown="启用" {
                  disable-tunnel: [w8943 w8946] -> w8938
                  disable-tunnel: [w8941 w8946] -> w8936
                  disable-tunnel: w8935 -> [w8940 _]
                  frame Disabled {
                    n3450 = Unbundle By Name(w8940) -> ("单体电压过低"=w8939:dbl)
                    n3451 = call "输入分辨率计算-EV05.vi"("1字节?"=FALSE, "数值"=w8939, "偏移量"=0.0, "分辨率"=0.001) -> ("低字节"=w8941:dbl, "高字节1"=w8943:dbl)  [unwired: 1 in, 5 out]
                  }
                  frame Enabled {
                    w8946 = 255 ("高字节1")
                  }
                }
                n3452 = Build Array(w8938, w8936) -> (w8937:i32[])
              }
              frame 9 {
                # "充电电流过高"
                n3453 = disable-structure shown="启用" {
                  disable-tunnel: [w8955 w8958] -> w8950
                  disable-tunnel: [w8953 w8958] -> w8948
                  disable-tunnel: w8947 -> [w8952 _]
                  frame Disabled {
                    n3454 = Unbundle By Name(w8952) -> ("充电电流过高"=w8951:dbl)
                    n3455 = call "输入分辨率计算-EV05.vi"("1字节?"=FALSE, "数值"=w8951, "偏移量"=-3000.0, "分辨率"=0.1) -> ("低字节"=w8953:dbl, "高字节1"=w8955:dbl)  [unwired: 1 in, 5 out]
                  }
                  frame Enabled {
                    w8958 = 255 ("高字节1")
                  }
                }
                n3456 = Build Array(w8950, w8948) -> (w8949:i32[])
              }
              frame 10 {
                # "放电电流过高"
                n3457 = disable-structure shown="启用" {
                  disable-tunnel: [w8967 w8970] -> w8962
                  disable-tunnel: [w8965 w8970] -> w8960
                  disable-tunnel: w8959 -> [w8964 _]
                  frame Disabled {
                    n3458 = Unbundle By Name(w8964) -> ("放电电流过高"=w8963:dbl)
                    n3459 = call "输入分辨率计算-EV05.vi"("1字节?"=FALSE, "数值"=w8963, "偏移量"=-3000.0, "分辨率"=0.1) -> ("低字节"=w8965:dbl, "高字节1"=w8967:dbl)  [unwired: 1 in, 5 out]
                  }
                  frame Enabled {
                    w8970 = 255 ("高字节1")
                  }
                }
                n3460 = Build Array(w8962, w8960) -> (w8961:i32[])
              }
              frame 11 {
                # "单组温度不均衡"
                n3461 = disable-structure shown="启用" {
                  disable-tunnel: [w8976 255 ("高字节1")] -> w8973
                  disable-tunnel: w8971 -> [w8975 _]
                  frame Enabled {
                    n3462 = Unbundle By Name(w8975) -> ("单组温度不均衡"=w8974:dbl)
                    n3463 = call "输入分辨率计算-EV05.vi"("1字节?"=TRUE, "数值"=w8974, "分辨率"=1.0) -> ("高字节1"=w8976:dbl)  [unwired: 2 in, 6 out]
                  }
                  frame Disabled {
                  }
                }
                n3464 = Build Array(w8973) -> (w8972:dbl[])
              }
              frame 12 {
                # "SOC过高"
                n3465 = Unbundle By Name(w8984) -> ("SOC过高"=w8983:dbl)
                n3466 = call "输入分辨率计算-EV05.vi"("1字节?"=FALSE, "数值"=w8983, "偏移量"=0.0, "分辨率"=0.1) -> ("低字节"=w8985:dbl, "高字节1"=w8986:dbl)  [unwired: 1 in, 5 out]
                n3467 = call "二进制解析-8.6.vi"("索引"=4, "数值"=w8986) -> ("低位子数组"=w8989:i32[])  [unwired: 3 out]
                n3468 = call "二进制解析-8.6.vi"("索引"=4, "数值"=w8985) -> ("低位子数组"=w8981:i32[], "高位子数组"=w8988:i32[])  [unwired: 2 out]
                n3469 = Insert Into Array(array=w8989, new element=w8988) -> (w8987:i32[])  [unwired: 1 in]
                n3470 = call "数值二进制转十进制-8.6.vi"("子数组"=w8987) -> ("十进制数值"=w8982:i32)  [unwired: 4 out]
                n3471 = disable-structure shown="启用" {
                  disable-tunnel: w8982 -> [w8997 _]
                  disable-tunnel: [w8997 255 ("高字节1")] -> w8980
                  disable-tunnel: w8981 -> [w8996 _]
                  disable-tunnel: [w8996 i32[] [] ("低位子数组 29")] -> _
                  frame Disabled {
                  }
                  frame Enabled {
                  }
                }
                n3472 = Build Array(w8980, w8980) -> (w8993:i32[])
              }
              frame 13 {
                # "SOC过低"
                n3473 = Unbundle By Name(w9005) -> ("SOC过低"=w9004:dbl)
                n3474 = call "输入分辨率计算-EV05.vi"("1字节?"=FALSE, "数值"=w9004, "偏移量"=0.0, "分辨率"=0.1) -> ("低字节"=w9002:dbl, "高字节1"=w9003:dbl)  [unwired: 1 in, 5 out]
                n3475 = call "二进制解析-8.6.vi"("索引"=4, "数值"=w9003) -> ("低位子数组"=w9001:i32[])  [unwired: 3 out]
                n3476 = disable-structure shown="启用" {
                  disable-tunnel: w9002 -> [w9012 _]
                  disable-tunnel: [w9012 255 ("高字节1")] -> w9000
                  disable-tunnel: w9001 -> [w9011 _]
                  disable-tunnel: [w9011 i32[] [] ("低位子数组")] -> _
                  frame Disabled {
                    (unwired) i32[] [] ("低位子数组 4")
                  }
                  frame Enabled {
                  }
                }
                n3477 = Build Array(w9000, w9000) -> (w9008:i32[])
              }
              frame 14 {
                # "内阻过大"
                n3478 = disable-structure shown="启用" {
                  disable-tunnel: w9017 -> [w9022 _]
                  disable-tunnel: [w9018 255 ("高字节1")] -> w9015
                  frame Disabled {
                    n3479 = Unbundle By Name(w9022) -> ("内阻过大"=w9021:dbl)
                    n3480 = call "输入分辨率计算-EV05.vi"("1字节?"=TRUE, "数值"=w9021, "分辨率"=0.1) -> ("高字节1"=w9018:dbl)  [unwired: 2 in, 6 out]
                  }
                  frame Enabled {
                  }
                }
                n3481 = Build Array(w9015) -> (w9016:i32[])
              }
              frame 15 {
                # "极柱温度过高"
                n3482 = disable-structure shown="启用" {
                  disable-tunnel: w9026 -> [w9032 _]
                  disable-tunnel: [w9028 255 ("高字节1")] -> w9024
                  frame Disabled {
                    n3483 = Unbundle By Name(w9032) -> ("极柱温度过高"=w9031:dbl)
                    n3484 = call "输入分辨率计算-EV05.vi"("1字节?"=TRUE, "数值"=w9031, "偏移量"=-40.0, "分辨率"=1.0) -> ("高字节1"=w9028:dbl)  [unwired: 1 in, 6 out]
                  }
                  frame Enabled {
                  }
                }
                n3485 = Build Array(w9024) -> (w9025:i32[])
              }
              frame 16 {
                # "SOH过低"
                n3486 = disable-structure shown="启用" {
                  disable-tunnel: [w9049 w9057] -> w9036
                  disable-tunnel: w9035 -> [w9046 _]
                  disable-tunnel: [w9038 w9057] -> w9034
                  frame Disabled {
                    n3487 = Unbundle By Name(w9046) -> ("SOH过低"=w9045:dbl)
                    n3488 = call "输入分辨率计算-EV05.vi"("1字节?"=FALSE, "数值"=w9045, "偏移量"=0.0, "分辨率"=0.1) -> ("低字节"=w9047:dbl, "高字节1"=w9048:dbl)  [unwired: 1 in, 5 out]
                    n3489 = call "二进制解析-8.6.vi"("索引"=4, "数值"=w9048) -> ("低位子数组"=w9051:i32[])  [unwired: 3 out]
                    n3490 = call "二进制解析-8.6.vi"("索引"=4, "数值"=w9047) -> ("低位子数组"=w9040:i32[], "高位子数组"=w9050:i32[])  [unwired: 2 out]
                    n3491 = call "二进制解析-8.6.vi"("索引"=4, "数值"=0) -> ("低位子数组"=w9041:i32[])  [unwired: 3 out]
                    n3492 = Insert Into Array(array=w9051, new element=w9050) -> (w9044:i32[])  [unwired: 1 in]
                    n3493 = Insert Into Array(array=w9040, new element=w9041) -> (w9039:i32[])  [unwired: 1 in]
                    n3494 = call "数值二进制转十进制-8.6.vi"("子数组"=w9044) -> ("十进制数值"=w9049:i32)  [unwired: 4 out]
                    n3495 = call "数值二进制转十进制-8.6.vi"("子数组"=w9039) -> ("十进制数值"=w9038:i32)  [unwired: 4 out]
                  }
                  frame Enabled {
                    w9057 = 255 ("高字节1")
                  }
                }
                n3496 = Build Array(w9036, w9034) -> (w9037:i32[])
              }
            }
            n3497 = Insert Into Array(array=w8843, new element=w8844) -> (w8842:dbl[])  [unwired: 1 in]
          }
          n3498 = Build Array(w8839) -> (w8838:dbl[][])
          n3499 = Build Array("二级故障阀值") -> (w8829:string[])
        }
        frame "单组温度不均衡(3)" {
          n3500 = Unbundle By Name(w9063) -> ("一级故障 3"=w9064:refnum<vi>)
          n3501 = property class="Clust (严格)"(reference=w9064) -> ("Value"=w9062:T4)  [unwired: 1 in, 2 out]
          n3502 = for {
            N: 17 -> [_]
            tunnel: w9062 -> [w9074]
            shift-right: [w9071] -> w9068
            shift-left: dbl[] [] -> [w9072]
            i -> [w9075]
            n3503 = case shown="11" w9075 {
              tunnel: w9074 -> [w9076 w9087 w9098 w9108 w9118 w9128 w9140 w9152 w9164 w9176 w9188 w9200 w9213 w9234 w9246 w9255 w9264]
              tunnel: [w9077 w9088 w9099 w9109 w9119 w9130 w9142 w9154 w9166 w9178 w9190 w9201 w9222 w9237 w9245 w9254 w9266] -> w9073
              frame 0, Default {
                # "总电压过高"
                n3504 = disable-structure shown="启用" {
                  disable-tunnel: [w9083 w9086] -> w9079
                  disable-tunnel: [w9082 w9086] -> w9078
                  disable-tunnel: w9076 -> [w9081 _]
                  frame Disabled {
                    n3505 = Unbundle By Name(w9081) -> ("总电压过高"=w9080:dbl)
                    n3506 = call "输入分辨率计算-EV05.vi"("1字节?"=FALSE, "数值"=w9080, "分辨率"=0.1) -> ("低字节"=w9083:dbl, "高字节1"=w9082:dbl)  [unwired: 2 in, 5 out]
                  }
                  frame Enabled {
                    w9086 = 255 ("高字节1")
                  }
                }
                n3507 = Build Array(w9078, w9079) -> (w9077:i32[])
              }
              frame 1 {
                # "总电压过低"
                n3508 = disable-structure shown="启用" {
                  disable-tunnel: [w9094 w9097] -> w9090
                  disable-tunnel: [w9093 w9097] -> w9089
                  disable-tunnel: w9087 -> [w9092 _]
                  frame Disabled {
                    n3509 = Unbundle By Name(w9092) -> ("总电压过低"=w9091:dbl)
                    n3510 = call "输入分辨率计算-EV05.vi"("1字节?"=FALSE, "数值"=w9091, "分辨率"=0.1) -> ("低字节"=w9094:dbl, "高字节1"=w9093:dbl)  [unwired: 2 in, 5 out]
                  }
                  frame Enabled {
                    w9097 = 255 ("高字节1")
                  }
                }
                n3511 = Build Array(w9089, w9090) -> (w9088:i32[])
              }
              frame 2 {
                # "温度过高"
                n3512 = disable-structure shown="启用" {
                  disable-tunnel: [w9104 255 ("高字节1")] -> w9100
                  disable-tunnel: w9098 -> [w9102 _]
                  frame Disabled {
                    n3513 = Unbundle By Name(w9102) -> ("温度过高"=w9101:dbl)
                    n3514 = call "输入分辨率计算-EV05.vi"("1字节?"=TRUE, "数值"=w9101, "偏移量"=-40.0, "分辨率"=1.0) -> ("高字节1"=w9104:dbl)  [unwired: 1 in, 6 out]
                  }
                  frame Enabled {
                  }
                }
                n3515 = Build Array(w9100) -> (w9099:i32[])
              }
              frame 3 {
                # "温度过低"
                n3516 = disable-structure shown="启用" {
                  disable-tunnel: [w9114 255 ("高字节1")] -> w9110
                  disable-tunnel: w9108 -> [w9112 _]
